vi "Try It.vi"(8 "error in":errorcluster, 11 "Demo":refnum<class "Demo.lvclass">) -> (0 "error out":errorcluster)   [LabVIEW 2025]
uses:
  Demo_class/Demo.lvclass
  Demo_class/Demo.lvclass/Demo.ctl
  Demo_class/Get VI.vi
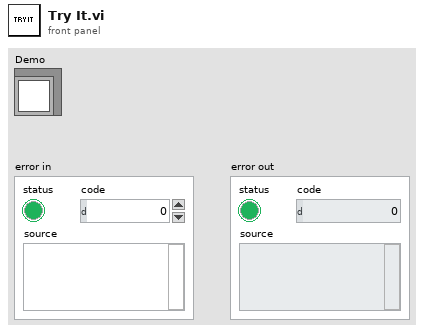
[diagram p1: front panel]
types:
  T1 = enum32{"Invalid", "Standard", "Closed", "Hidden", "Minimized", "Maximized"}
  T2 = typedef "LVRectTypeDef.ctl" = cluster{"Left":i16, "Top":i16, "Right":i16, "Bottom":i16}
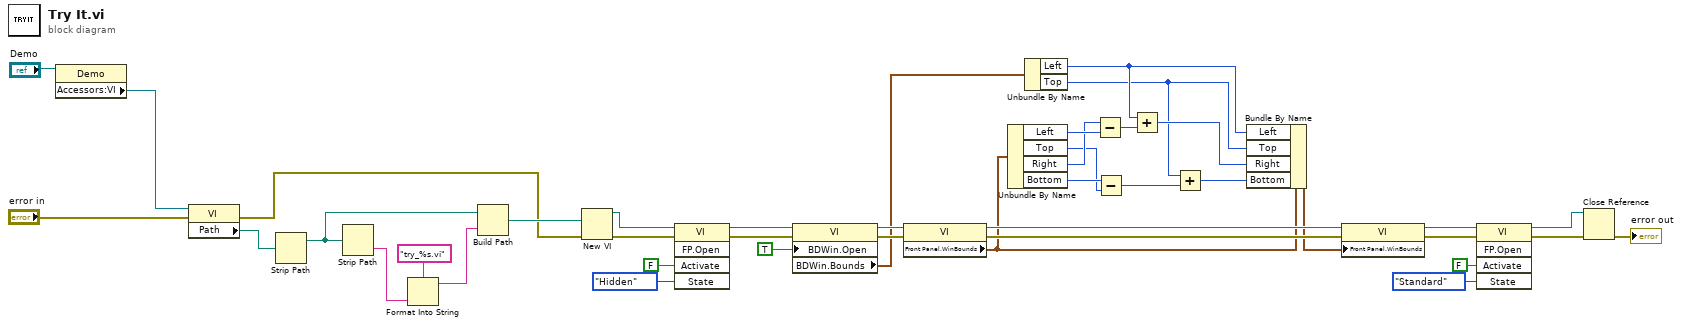
[diagram p0: block diagram]
diagram:
  n1 = property class="Demo"(reference="Demo") -> ("Accessors:VI"=w39:refnum<vi>)  [unwired: 1 in, 2 out]
  n2 = property class="VI"(reference=w39, error in="error in") -> (error out=w32:errorcluster, "Path"=w38:path)  [unwired: 1 out]
  n3 = Strip Path(path=w38) -> (stripped path=w37:path)  [unwired: 1 out]
  n4 = Strip Path(path=w37) -> (name=w35:string)  [unwired: 1 out]
  n5 = Format Into String(format string="try_%s.vi", w35) -> (resulting string=w34:string)  [unwired: 2 in, 1 out]
  n6 = Build Path(base path=w37, name or relative path=w34) -> (appended path=w33:path)
  n7 = New VI(8:w32, 10:w33) -> (0:w31:errorcluster, 3:w26:refnum<vi>)  [unwired: 5 in]
  n8 = invoke class="VI" method="FP.Open"(reference=w26, error in=w31, "Activate"=FALSE ("Activate?"), "State"=T1."Hidden") -> (reference out=w25:refnum<vi>, error out=w27:errorcluster)  [unwired: 1 in, 3 out]
  n9 = property class="VI"(reference=w25, error in=w27, "BDWin.Open"=TRUE ("Block Diagram Window:Open")) -> (reference out=w21:refnum<vi>, error out=w29:errorcluster, "BDWin.Bounds"=w16:T2)
  n10 = property class="VI"(reference=w21, error in=w29) -> (reference out=w19:refnum<vi>, error out=w22:errorcluster, "Front Panel.WinBounds"=w18:T2)
  n11 = Unbundle By Name(w18) -> ("Left"=w15:i16, "Top"=w9:i16, "Right"=w14:i16, "Bottom"=w10:i16)
  n12 = Unbundle By Name(w16) -> ("Left"=w12:i16, "Top"=w7:i16)
  n13 = Subtract(x=w14, y=w15) -> (x-y=w13:i16)
  n14 = Subtract(x=w10, y=w9) -> (x-y=w8:i16)
  n15 = Add(x=w12, y=w13) -> (x+y=w11:i16)
  n16 = Add(x=w7, y=w8) -> (x+y=w6:i16)
  n17 = Bundle By Name(cluster=w18, "Left"=w12, "Top"=w7, "Right"=w11, "Bottom"=w6) -> (w17:T2)
  n18 = property class="VI"(reference=w19, error in=w22, "Front Panel.WinBounds"=w17) -> (reference out=w4:refnum<vi>, error out=w20:errorcluster)
  n19 = invoke class="VI" method="FP.Open"(reference=w4, error in=w20, "Activate"=FALSE ("Activate?"), "State"=T1."Standard") -> (reference out=w3:refnum<vi>, error out=w5:errorcluster)  [unwired: 1 in, 3 out]
  n20 = Close Reference(reference=w3, error in (no error)=w5) -> (error out=→"error out":errorcluster)
